vi "ChangeData.vi"(2 "data":string="\"§¶C54ÍÀì6#D\u000b\u00033Ã\u0014ð©À\u0002°B\u0000\u0000\u0000\u0000\u0000\u0000\u0000\u0000\u0006\u0000\u0000\u0000\u0000\u0000\u0010\u0000", 3 "type":string="é\u0003") -> (0 "out":string[][](array[string]), 1 "Contents":string)   [LabVIEW 2018]
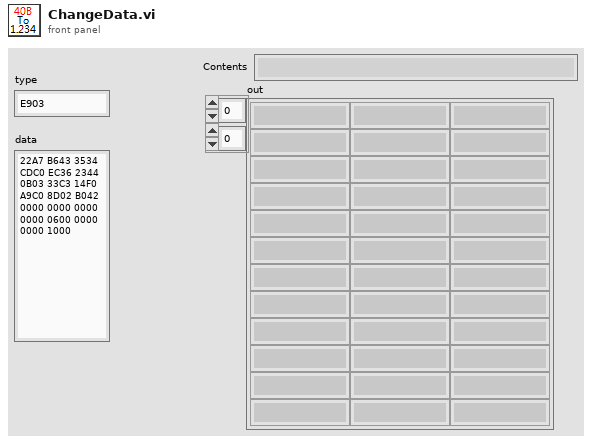
[diagram p1: front panel]
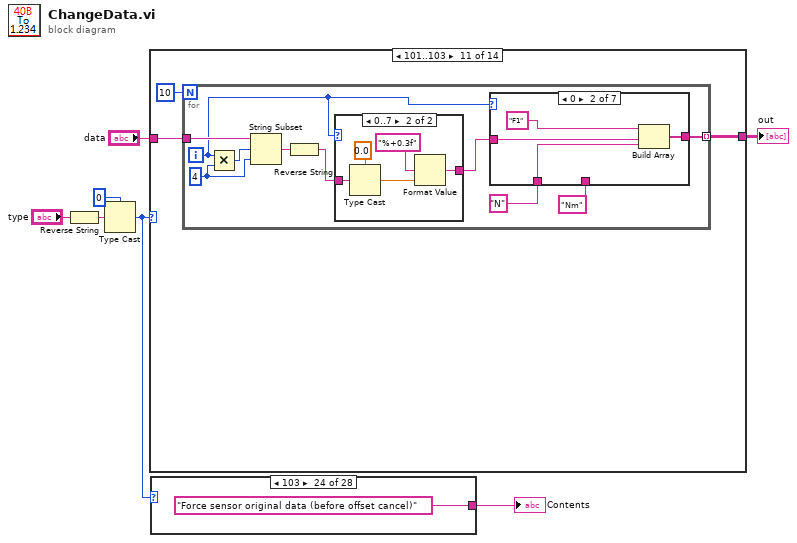
[diagram p0: block diagram]
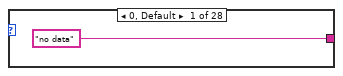
[diagram p2: hidden frame]
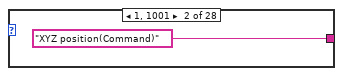
[diagram p3: hidden frame]
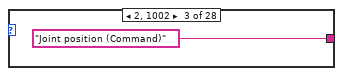
[diagram p4: hidden frame]
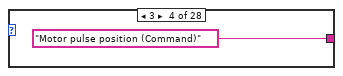
[diagram p5: hidden frame]
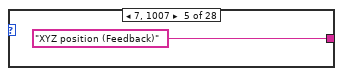
[diagram p6: hidden frame]
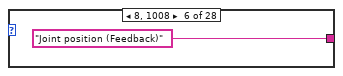
[diagram p7: hidden frame]
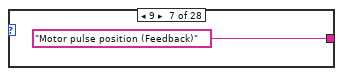
[diagram p8: hidden frame]
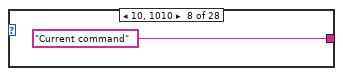
[diagram p9: hidden frame]
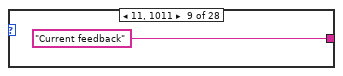
[diagram p10: hidden frame]
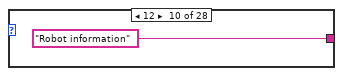
[diagram p11: hidden frame]
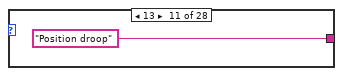
[diagram p12: hidden frame]
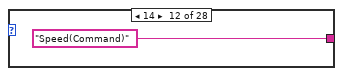
[diagram p13: hidden frame]
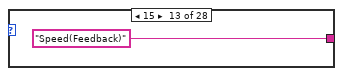
[diagram p14: hidden frame]
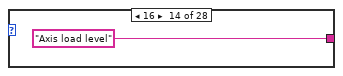
[diagram p15: hidden frame]
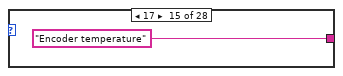
[diagram p16: hidden frame]
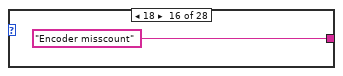
[diagram p17: hidden frame]
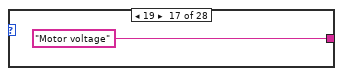
[diagram p18: hidden frame]
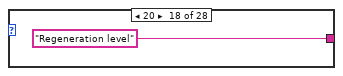
[diagram p19: hidden frame]
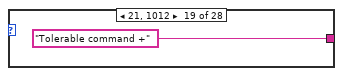
[diagram p20: hidden frame]
diagram:
  n1 = Reverse String(1:"type") -> (0:w7:string)
  n2 = Type Cast(type=u16 0, x=w7) -> (*(type *) &x=w3:u16)
  n3 = case shown="101..103" w3 {
    tunnel: "data" -> [_ w10 w81 w133 w185 w239 w299 w394 w446 w498 w530 w575 w646 w698]
    tunnel: [string[][] [] w9 w80 w132 w184 w238 w322 w393 w445 w497 w529 w574 w645 w697] -> w1
    frame 0, Default {
    }
    frame 1, 7 {
      n4 = for {
        N: 10 -> [_]
        tunnel: w10 -> [w21]
        tunnel: [w17] -> w9 mode=indexing
        i -> [w14]
        w18 = 4
        n5 = Multiply(x=w14, y=w18) -> (x*y=w20:i32)
        n6 = String Subset(string=w21, offset (0)=w20, length (rest)=w18) -> (substring=w19:string)
        n7 = Reverse String(1:w19) -> (0:w16:string)
        n8 = case shown="0..7" w14 {
          tunnel: w16 -> [w22 w24 w31 w36]
          tunnel: [w22 w23 w28 w33] -> w15
          frame -1, Default {
          }
          frame 0..7 {
            n9 = Type Cast(type=sgl 0.0, x=w24) -> (*(type *) &x=w26:sgl)
            n10 = Format Value(format string="%+0.3f", value (0)=w26) -> (output string=w23:string)  [unwired: 1 in]
          }
          frame 8 {
            n11 = Type Cast(type=u32 0, x=w31) -> (*(type *) &x=w30:u32)
            n12 = Format Value(format string="B%08b" ("格式字符串"), value (0)=w30) -> (output string=w28:string)  [unwired: 1 in]
          }
          frame 9 {
            n13 = Type Cast(type=u32 0, x=w36) -> (*(type *) &x=w35:u32)
            n14 = Format Value(format string="H%08x" ("格式字符串"), value (0)=w35) -> (output string=w33:string)  [unwired: 1 in]
          }
        }
        n15 = case shown="8" w14 {
          tunnel: w15 -> [_ w42 w46 w50 w54 w58 w62 w66 w70 w74 w78]
          tunnel: [w38 w41 w45 w49 w53 w57 w61 w64 w68 w72 w76] -> w17
          tunnel: "mm" -> [_ w40 w44 w48 _ _ _ _ _ _ _]
          tunnel: "rad" -> [_ _ _ _ w52 w56 w60 _ _ _ _]
          frame -1, Default {
            w39 = ""
            n16 = Build Array(w39, w39, w39) -> (w38:string[])
          }
          frame 0 {
            n17 = Build Array("X", w42, w40) -> (w41:string[])
          }
          frame 1 {
            n18 = Build Array("Y", w46, w44) -> (w45:string[])
          }
          frame 2 {
            n19 = Build Array("Z", w50, w48) -> (w49:string[])
          }
          frame 3 {
            n20 = Build Array("A", w54, w52) -> (w53:string[])
          }
          frame 4 {
            n21 = Build Array("B", w58, w56) -> (w57:string[])
          }
          frame 5 {
            n22 = Build Array("C", w62, w60) -> (w61:string[])
          }
          frame 6 {
            n23 = Build Array("L1", w66, "") -> (w64:string[])
          }
          frame 7 {
            n24 = Build Array("L2", w70, "") -> (w68:string[])
          }
          frame 8 {
            n25 = Build Array("FL1", w74, "") -> (w72:string[])
          }
          frame 9 {
            n26 = Build Array("FL2", w78, "") -> (w76:string[])
          }
        }
      }
    }
    frame 2, 8 {
      n27 = for {
        N: 10 -> [_]
        tunnel: w81 -> [w91]
        tunnel: [w87] -> w80 mode=indexing
        i -> [w84]
        w88 = 4
        n28 = Multiply(x=w84, y=w88) -> (x*y=w90:i32)
        n29 = String Subset(string=w91, offset (0)=w90, length (rest)=w88) -> (substring=w89:string)
        n30 = Reverse String(1:w89) -> (0:w86:string)
        n31 = case shown="0..7" w84 {
          tunnel: w86 -> [_ w94]
          tunnel: ["" w93] -> w85
          frame -1, Default {
          }
          frame 0..7 {
            n32 = Type Cast(type=sgl 0.0, x=w94) -> (*(type *) &x=w96:sgl)
            n33 = Format Value(format string="%+0.3f", value (0)=w96) -> (output string=w93:string)  [unwired: 1 in]
          }
        }
        n34 = case shown="0" w84 {
          tunnel: w85 -> [_ w102 w106 w110 w114 w118 w122 w126 w130]
          tunnel: [w98 w101 w107 w109 w113 w117 w121 w125 w129] -> w87
          tunnel: "rad" -> [_ w100 w104 w108 w112 w116 w120 w124 w128]
          frame -1, Default {
            w99 = ""
            n35 = Build Array(w99, w99, w99) -> (w98:string[])
          }
          frame 0 {
            n36 = Build Array("J1", w102, w100) -> (w101:string[])
          }
          frame 1 {
            n37 = Build Array("J2", w106, w104) -> (w107:string[])
          }
          frame 2 {
            n38 = Build Array("J3", w110, w108) -> (w109:string[])
          }
          frame 3 {
            n39 = Build Array("J4", w114, w112) -> (w113:string[])
          }
          frame 4 {
            n40 = Build Array("J5", w118, w116) -> (w117:string[])
          }
          frame 5 {
            n41 = Build Array("J6", w122, w120) -> (w121:string[])
          }
          frame 6 {
            n42 = Build Array("J7", w126, w124) -> (w125:string[])
          }
          frame 7 {
            n43 = Build Array("J8", w130, w128) -> (w129:string[])
          }
        }
      }
    }
    frame 3, 9, 13, 18 {
      n44 = for {
        N: 10 -> [_]
        tunnel: w133 -> [w143]
        tunnel: [w139] -> w132 mode=indexing
        i -> [w136]
        w140 = 4
        n45 = Multiply(x=w136, y=w140) -> (x*y=w142:i32)
        n46 = String Subset(string=w143, offset (0)=w142, length (rest)=w140) -> (substring=w141:string)
        n47 = Reverse String(1:w141) -> (0:w138:string)
        n48 = case shown="0..7" w136 {
          tunnel: w138 -> [_ w146]
          tunnel: ["" w145] -> w137
          frame -1, Default {
          }
          frame 0..7 {
            n49 = Type Cast(type=0, x=w146) -> (*(type *) &x=w148:i32)
            n50 = Format Value(format string="%+d", value (0)=w148) -> (output string=w145:string)  [unwired: 1 in]
          }
        }
        n51 = case shown="0" w136 {
          tunnel: w137 -> [_ w154 w158 w162 w166 w170 w174 w178 w182]
          tunnel: [w150 w153 w157 w161 w165 w169 w173 w177 w181] -> w139
          tunnel: "pulse" -> [_ w152 w156 w160 w164 w168 w172 w176 w180]
          frame -1, Default {
            w151 = ""
            n52 = Build Array(w151, w151, w151) -> (w150:string[])
          }
          frame 0 {
            n53 = Build Array("M1", w154, w152) -> (w153:string[])
          }
          frame 1 {
            n54 = Build Array("M2", w158, w156) -> (w157:string[])
          }
          frame 2 {
            n55 = Build Array("M3", w162, w160) -> (w161:string[])
          }
          frame 3 {
            n56 = Build Array("M4", w166, w164) -> (w165:string[])
          }
          frame 4 {
            n57 = Build Array("M5", w170, w168) -> (w169:string[])
          }
          frame 5 {
            n58 = Build Array("M6", w174, w172) -> (w173:string[])
          }
          frame 6 {
            n59 = Build Array("M7", w178, w176) -> (w177:string[])
          }
          frame 7 {
            n60 = Build Array("M8", w182, w180) -> (w181:string[])
          }
        }
      }
    }
    frame 10, 11, 21..23, 111..113 {
      n61 = for {
        N: 10 -> [_]
        tunnel: w185 -> [w195]
        tunnel: [w191] -> w184 mode=indexing
        i -> [w188]
        w192 = 4
        n62 = Multiply(x=w188, y=w192) -> (x*y=w194:i32)
        n63 = String Subset(string=w195, offset (0)=w194, length (rest)=w192) -> (substring=w193:string)
        n64 = Reverse String(1:w193) -> (0:w190:string)
        n65 = case shown="0..7" w188 {
          tunnel: w190 -> [_ w201]
          tunnel: ["" w200] -> w189
          frame -1, Default {
          }
          frame 0..7 {
            n66 = Type Cast(type=0, x=w201) -> (*(type *) &x=w199:i32)
            n67 = Divide(x=w199, y=10.0) -> (x/y=w197:dbl)
            n68 = Format Value(format string="%0.1f", value (0)=w197) -> (output string=w200:string)  [unwired: 1 in]
          }
        }
        n69 = case shown="0" w188 {
          tunnel: w189 -> [_ w208 w212 w216 w220 w224 w228 w232 w236]
          tunnel: [w204 w207 w211 w215 w219 w223 w227 w231 w235] -> w191
          tunnel: "%" -> [_ w206 w210 w214 w218 w222 w226 w230 w234]
          frame -1, Default {
            w205 = ""
            n70 = Build Array(w205, w205, w205) -> (w204:string[])
          }
          frame 0 {
            n71 = Build Array("M1", w208, w206) -> (w207:string[])
          }
          frame 1 {
            n72 = Build Array("M2", w212, w210) -> (w211:string[])
          }
          frame 2 {
            n73 = Build Array("M3", w216, w214) -> (w215:string[])
          }
          frame 3 {
            n74 = Build Array("M4", w220, w218) -> (w219:string[])
          }
          frame 4 {
            n75 = Build Array("M5", w224, w222) -> (w223:string[])
          }
          frame 5 {
            n76 = Build Array("M6", w228, w226) -> (w227:string[])
          }
          frame 6 {
            n77 = Build Array("M7", w232, w230) -> (w231:string[])
          }
          frame 7 {
            n78 = Build Array("M8", w236, w234) -> (w235:string[])
          }
        }
      }
    }
    frame 14, 15 {
      n79 = for {
        N: 10 -> [_]
        tunnel: w239 -> [w249]
        tunnel: [w245] -> w238 mode=indexing
        i -> [w242]
        w246 = 4
        n80 = Multiply(x=w242, y=w246) -> (x*y=w248:i32)
        n81 = String Subset(string=w249, offset (0)=w248, length (rest)=w246) -> (substring=w247:string)
        n82 = Reverse String(1:w247) -> (0:w244:string)
        n83 = case shown="0..7" w242 {
          tunnel: w244 -> [_ w253]
          tunnel: ["" w252] -> w243
          frame -1, Default {
          }
          frame 0..7 {
            n84 = Type Cast(type=0, x=w253) -> (*(type *) &x=w251:i32)
            n85 = Format Value(format string="%d", value (0)=w251) -> (output string=w252:string)  [unwired: 1 in]
          }
        }
        n86 = case shown="0" w242 {
          tunnel: w243 -> [_ w260 w264 w268 w272 w276 w280 w284 w288]
          tunnel: [w256 w259 w263 w267 w271 w275 w279 w283 w287] -> w245
          tunnel: "rpm" -> [_ w258 w262 w266 w270 w274 w278 w282 w286]
          frame -1, Default {
            w257 = ""
            n87 = Build Array(w257, w257, w257) -> (w256:string[])
          }
          frame 0 {
            n88 = Build Array("M1", w260, w258) -> (w259:string[])
          }
          frame 1 {
            n89 = Build Array("M2", w264, w262) -> (w263:string[])
          }
          frame 2 {
            n90 = Build Array("M3", w268, w266) -> (w267:string[])
          }
          frame 3 {
            n91 = Build Array("M4", w272, w270) -> (w271:string[])
          }
          frame 4 {
            n92 = Build Array("M5", w276, w274) -> (w275:string[])
          }
          frame 5 {
            n93 = Build Array("M6", w280, w278) -> (w279:string[])
          }
          frame 6 {
            n94 = Build Array("M7", w284, w282) -> (w283:string[])
          }
          frame 7 {
            n95 = Build Array("M8", w288, w286) -> (w287:string[])
          }
        }
      }
    }
    frame 12 {
      n96 = for {
        N: 5 -> [_]
        tunnel: w299 -> [w370]
        tunnel: [w366] -> w324 mode=indexing
        i -> [w363]
        w367 = 4
        n97 = Multiply(x=w363, y=w367) -> (x*y=w369:i32)
        n98 = String Subset(string=w370, offset (0)=w369, length (rest)=w367) -> (substring=w368:string)
        n99 = Reverse String(1:w368) -> (0:w365:string)
        n100 = Type Cast(type=0, x=w365) -> (*(type *) &x=w360:i32)
        n101 = Format Value(format string="%d", value (0)=w360) -> (output string=w364:string)  [unwired: 1 in]
        n102 = case shown="0" w363 {
          tunnel: w364 -> [_ w375 w379 w383 w387 w391]
          tunnel: [w371 w374 w378 w382 w386 w390] -> w366
          frame -1, Default {
            w372 = ""
            n103 = Build Array(w372, w372, w372) -> (w371:string[])
          }
          frame 0 {
            n104 = Build Array("Tool point speed(feedback)", w375, "mm/s") -> (w374:string[])
          }
          frame 1 {
            n105 = Build Array("Remaining distance(feedback)", w379, "mm") -> (w378:string[])
          }
          frame 2 {
            n106 = Build Array("Tool point speed(Command)", w383, "mm/s") -> (w382:string[])
          }
          frame 3 {
            n107 = Build Array("Remaining distance(Command)", w387, "mm") -> (w386:string[])
          }
          frame 4 {
            n108 = Build Array("Gap of command and feedback", w391, "") -> (w390:string[])
          }
        }
      }
      n109 = String Subset(string=w299, offset (0)=20 ("偏移量(0)"), length (rest)=6 ("长度（剩余）")) -> (substring=w326:string)
      n110 = String Subset(string=w299, offset (0)=26 ("偏移量(0)"), length (rest)=6 ("长度（剩余）")) -> (substring=w319:string)
      n111 = String Subset(string=w299, offset (0)=32 ("偏移量(0)"), length (rest)=2 ("长度（剩余）")) -> (substring=w312:string)
      n112 = String Subset(string=w299, offset (0)=36 ("偏移量(0)"), length (rest)=4 ("长度（剩余）")) -> (substring=w298:string)
      n113 = for {
        N: 3 -> [_]
        tunnel: w326 -> [w334]
        tunnel: [w330] -> w323 mode=indexing
        i -> [w332]
        w333 = 2
        n114 = Multiply(x=w332, y=w333) -> (x*y=w336:i32)
        n115 = String Subset(string=w334, offset (0)=w336, length (rest)=w333) -> (substring=w337:string)
        n116 = Reverse String(1:w337) -> (0:w338:string)
        n117 = Type Cast(type=i16 0, x=w338) -> (*(type *) &x=w340:i16)
        n118 = Format Value(format string="%d", value (0)=w340) -> (output string=w331:string)  [unwired: 1 in]
        n119 = case shown="2" w332 {
          tunnel: w331 -> [_ w345 w348 w358]
          tunnel: [w341 w343 w349 w356] -> w330
          frame -1, Default {
            w342 = ""
            n120 = Build Array(w342, w342, w342) -> (w341:string[])
          }
          frame 0 {
            n121 = Build Array("Transport factor (command)", w345, "") -> (w343:string[])
          }
          frame 1 {
            n122 = case shown="\"假\", 默认" w348 {
              tunnel: ["" "Stopped" "Accelerating" "Constant speed" "Decelerating"] -> w347
              frame "假", Default {
              }
              frame "0" {
              }
              frame "1" {
              }
              frame "2" {
              }
              frame "3" {
              }
            }
            n123 = Build Array("Acceleration state(command)", w348, w347) -> (w349:string[])
          }
          frame 2 {
            n124 = Build Array("Step number( slot 1)", w358, "") -> (w356:string[])
          }
        }
      }
      n125 = Reverse String(1:w298) -> (0:w297:string)
      n126 = Reverse String(1:w319) -> (0:w316:string)
      n127 = Reverse String(1:w312) -> (0:w311:string)
      n128 = Type Cast(type=0, x=w297) -> (*(type *) &x=w295:i32)
      n129 = Type Cast(type=i16 0, x=w311) -> (*(type *) &x=w309:i16)
      n130 = Divide(x=w309, y=i16 10) -> (x/y=w307:dbl)
      n131 = Format Value(format string="%d", value (0)=w295) -> (output string=w291:string)  [unwired: 1 in]
      n132 = Format Value(format string="%0.1f", value (0)=w307) -> (output string=w303:string)  [unwired: 1 in]
      n133 = Build Array("Program name( slot 1)", w316, "") -> (w315:string[])
      n134 = Build Array("Monitoring counter", w291, "X 7.1ms") -> (w290:string[])
      n135 = Build Array("Controller temperature", w303, "℃") -> (w302:string[])
      n136 = Build Array (concatenate)(w324, w323, w315, w302, w290) -> (w322:string[][])
    }
    frame 16, 20 {
      n137 = for {
        N: 10 -> [_]
        tunnel: w394 -> [w404]
        tunnel: [w400] -> w393 mode=indexing
        i -> [w397]
        w401 = 4
        n138 = Multiply(x=w397, y=w401) -> (x*y=w403:i32)
        n139 = String Subset(string=w404, offset (0)=w403, length (rest)=w401) -> (substring=w402:string)
        n140 = Reverse String(1:w402) -> (0:w399:string)
        n141 = case shown="0..7" w397 {
          tunnel: w399 -> [_ w408]
          tunnel: ["" w407] -> w398
          frame -1, Default {
          }
          frame 0..7 {
            n142 = Type Cast(type=sgl 0.0, x=w408) -> (*(type *) &x=w406:sgl)
            n143 = Format Value(format string="%0.3f", value (0)=w406) -> (output string=w407:string)  [unwired: 1 in]
          }
        }
        n144 = case shown="0" w397 {
          tunnel: w398 -> [_ w415 w419 w423 w427 w431 w435 w439 w443]
          tunnel: [w411 w414 w418 w422 w426 w430 w434 w438 w442] -> w400
          tunnel: "%" -> [_ w413 w417 w421 w425 w429 w433 w437 w441]
          frame -1, Default {
            w412 = ""
            n145 = Build Array(w412, w412, w412) -> (w411:string[])
          }
          frame 0 {
            n146 = Build Array("M1", w415, w413) -> (w414:string[])
          }
          frame 1 {
            n147 = Build Array("M2", w419, w417) -> (w418:string[])
          }
          frame 2 {
            n148 = Build Array("M3", w423, w421) -> (w422:string[])
          }
          frame 3 {
            n149 = Build Array("M4", w427, w425) -> (w426:string[])
          }
          frame 4 {
            n150 = Build Array("M5", w431, w429) -> (w430:string[])
          }
          frame 5 {
            n151 = Build Array("M6", w435, w433) -> (w434:string[])
          }
          frame 6 {
            n152 = Build Array("M7", w439, w437) -> (w438:string[])
          }
          frame 7 {
            n153 = Build Array("M8", w443, w441) -> (w442:string[])
          }
        }
      }
    }
    frame 17 {
      n154 = for {
        N: 10 -> [_]
        tunnel: w446 -> [w456]
        tunnel: [w452] -> w445 mode=indexing
        i -> [w449]
        w453 = 4
        n155 = Multiply(x=w449, y=w453) -> (x*y=w455:i32)
        n156 = String Subset(string=w456, offset (0)=w455, length (rest)=w453) -> (substring=w454:string)
        n157 = Reverse String(1:w454) -> (0:w451:string)
        n158 = case shown="0..7" w449 {
          tunnel: w451 -> [_ w460]
          tunnel: ["" w459] -> w450
          frame -1, Default {
          }
          frame 0..7 {
            n159 = Type Cast(type=0, x=w460) -> (*(type *) &x=w458:i32)
            n160 = Format Value(format string="%d", value (0)=w458) -> (output string=w459:string)  [unwired: 1 in]
          }
        }
        n161 = case shown="0" w449 {
          tunnel: w450 -> [_ w467 w471 w475 w479 w483 w487 w491 w495]
          tunnel: [w463 w466 w470 w474 w478 w482 w486 w490 w494] -> w452
          tunnel: "℃" -> [_ w465 w469 w473 w477 w481 w485 w489 w493]
          frame -1, Default {
            w464 = ""
            n162 = Build Array(w464, w464, w464) -> (w463:string[])
          }
          frame 0 {
            n163 = Build Array("M1", w467, w465) -> (w466:string[])
          }
          frame 1 {
            n164 = Build Array("M2", w471, w469) -> (w470:string[])
          }
          frame 2 {
            n165 = Build Array("M3", w475, w473) -> (w474:string[])
          }
          frame 3 {
            n166 = Build Array("M4", w479, w477) -> (w478:string[])
          }
          frame 4 {
            n167 = Build Array("M5", w483, w481) -> (w482:string[])
          }
          frame 5 {
            n168 = Build Array("M6", w487, w485) -> (w486:string[])
          }
          frame 6 {
            n169 = Build Array("M7", w491, w489) -> (w490:string[])
          }
          frame 7 {
            n170 = Build Array("M8", w495, w493) -> (w494:string[])
          }
        }
      }
    }
    frame 19 {
      n171 = for {
        N: 10 -> [_]
        tunnel: w498 -> [w508]
        tunnel: [w504] -> w497 mode=indexing
        i -> [w501]
        w505 = 4
        n172 = Multiply(x=w501, y=w505) -> (x*y=w507:i32)
        n173 = String Subset(string=w508, offset (0)=w507, length (rest)=w505) -> (substring=w506:string)
        n174 = Reverse String(1:w506) -> (0:w503:string)
        n175 = case shown="0..2" w501 {
          tunnel: w503 -> [_ w512]
          tunnel: ["" w511] -> w502
          frame -1, Default {
          }
          frame 0..2 {
            n176 = Type Cast(type=0, x=w512) -> (*(type *) &x=w510:i32)
            n177 = Format Value(format string="%d", value (0)=w510) -> (output string=w511:string)  [unwired: 1 in]
          }
        }
        n178 = case shown="2" w501 {
          tunnel: w502 -> [_ w519 w523 w527]
          tunnel: [w515 w518 w522 w526] -> w504
          tunnel: "V" -> [_ w517 w521 w525]
          frame -1, Default {
            w516 = ""
            n179 = Build Array(w516, w516, w516) -> (w515:string[])
          }
          frame 0 {
            n180 = Build Array("Motor power voltage", w519, w517) -> (w518:string[])
          }
          frame 1 {
            n181 = Build Array("Motor power voltage(MAX)", w523, w521) -> (w522:string[])
          }
          frame 2 {
            n182 = Build Array("Motor power voltage(MIN)", w527, w525) -> (w526:string[])
          }
        }
      }
    }
    frame 101..103 {
      n183 = for {
        N: 10 -> [_]
        tunnel: w530 -> [w541]
        tunnel: [w537] -> w529 mode=indexing
        i -> [w534]
        w538 = 4
        n184 = Multiply(x=w534, y=w538) -> (x*y=w540:i32)
        n185 = String Subset(string=w541, offset (0)=w540, length (rest)=w538) -> (substring=w539:string)
        n186 = Reverse String(1:w539) -> (0:w536:string)
        n187 = case shown="0..7" w534 {
          tunnel: w536 -> [_ w545]
          tunnel: ["" w544] -> w535
          frame -1, Default {
          }
          frame 0..7 {
            n188 = Type Cast(type=0.0, x=w545) -> (*(type *) &x=w543:dbl)
            n189 = Format Value(format string="%+0.3f", value (0)=w543) -> (output string=w544:string)  [unwired: 1 in]
          }
        }
        n190 = case shown="0" w534 {
          tunnel: w535 -> [_ w552 w556 w560 w564 w568 w572]
          tunnel: [w548 w551 w555 w559 w563 w567 w571] -> w537
          tunnel: "N" -> [_ w550 w554 w558 _ _ _]
          tunnel: "Nm" -> [_ _ _ _ w562 w566 w570]
          frame -1, Default {
            w549 = ""
            n191 = Build Array(w549, w549, w549) -> (w548:string[])
          }
          frame 0 {
            n192 = Build Array("F1", w552, w550) -> (w551:string[])
          }
          frame 1 {
            n193 = Build Array("F2", w556, w554) -> (w555:string[])
          }
          frame 2 {
            n194 = Build Array("F3", w560, w558) -> (w559:string[])
          }
          frame 3 {
            n195 = Build Array("F4", w564, w562) -> (w563:string[])
          }
          frame 4 {
            n196 = Build Array("F5", w568, w566) -> (w567:string[])
          }
          frame 5 {
            n197 = Build Array("F6", w572, w570) -> (w571:string[])
          }
        }
      }
    }
    frame 1001, 1007 {
      n198 = for {
        N: 10 -> [_]
        tunnel: w575 -> [w586]
        tunnel: [w582] -> w574 mode=indexing
        i -> [w579]
        w583 = 4
        n199 = Multiply(x=w579, y=w583) -> (x*y=w585:i32)
        n200 = String Subset(string=w586, offset (0)=w585, length (rest)=w583) -> (substring=w584:string)
        n201 = Reverse String(1:w584) -> (0:w581:string)
        n202 = case shown="0..7" w579 {
          tunnel: w581 -> [w587 w589 w596 w601]
          tunnel: [w587 w588 w593 w598] -> w580
          frame -1, Default {
          }
          frame 0..7 {
            n203 = Type Cast(type=sgl 0.0, x=w589) -> (*(type *) &x=w591:sgl)
            n204 = Format Value(format string="%+0.3f", value (0)=w591) -> (output string=w588:string)  [unwired: 1 in]
          }
          frame 8 {
            n205 = Type Cast(type=u32 0, x=w596) -> (*(type *) &x=w595:u32)
            n206 = Format Value(format string="B%08b" ("格式字符串"), value (0)=w595) -> (output string=w593:string)  [unwired: 1 in]
          }
          frame 9 {
            n207 = Type Cast(type=u32 0, x=w601) -> (*(type *) &x=w600:u32)
            n208 = Format Value(format string="H%08x" ("格式字符串"), value (0)=w600) -> (output string=w598:string)  [unwired: 1 in]
          }
        }
        n209 = case shown="5" w579 {
          tunnel: w580 -> [_ w607 w611 w615 w619 w623 w627 w631 w635 w639 w643]
          tunnel: [w603 w606 w610 w614 w618 w622 w626 w629 w633 w637 w641] -> w582
          tunnel: "mm" -> [_ w605 w609 w613 _ _ _ _ _ _ _]
          tunnel: "deg" -> [_ _ _ _ w617 w621 w625 _ _ _ _]
          frame -1, Default {
            w604 = ""
            n210 = Build Array(w604, w604, w604) -> (w603:string[])
          }
          frame 0 {
            n211 = Build Array("X", w607, w605) -> (w606:string[])
          }
          frame 1 {
            n212 = Build Array("Y", w611, w609) -> (w610:string[])
          }
          frame 2 {
            n213 = Build Array("Z", w615, w613) -> (w614:string[])
          }
          frame 3 {
            n214 = Build Array("A", w619, w617) -> (w618:string[])
          }
          frame 4 {
            n215 = Build Array("B", w623, w621) -> (w622:string[])
          }
          frame 5 {
            n216 = Build Array("C", w627, w625) -> (w626:string[])
          }
          frame 6 {
            n217 = Build Array("L1", w631, "") -> (w629:string[])
          }
          frame 7 {
            n218 = Build Array("L2", w635, "") -> (w633:string[])
          }
          frame 8 {
            n219 = Build Array("FL1", w639, "") -> (w637:string[])
          }
          frame 9 {
            n220 = Build Array("FL2", w643, "") -> (w641:string[])
          }
        }
      }
    }
    frame 1002, 1008 {
      n221 = for {
        N: 10 -> [_]
        tunnel: w646 -> [w656]
        tunnel: [w652] -> w645 mode=indexing
        i -> [w649]
        w653 = 4
        n222 = Multiply(x=w649, y=w653) -> (x*y=w655:i32)
        n223 = String Subset(string=w656, offset (0)=w655, length (rest)=w653) -> (substring=w654:string)
        n224 = Reverse String(1:w654) -> (0:w651:string)
        n225 = case shown="0..7" w649 {
          tunnel: w651 -> [_ w659]
          tunnel: ["" w658] -> w650
          frame -1, Default {
          }
          frame 0..7 {
            n226 = Type Cast(type=sgl 0.0, x=w659) -> (*(type *) &x=w661:sgl)
            n227 = Format Value(format string="%+0.3f", value (0)=w661) -> (output string=w658:string)  [unwired: 1 in]
          }
        }
        n228 = case shown="3" w649 {
          tunnel: w650 -> [_ w667 w671 w675 w679 w683 w687 w691 w695]
          tunnel: [w663 w666 w672 w674 w678 w682 w686 w690 w694] -> w652
          tunnel: "deg" -> [_ w665 w669 w673 w677 w681 w685 w689 w693]
          frame -1, Default {
            w664 = ""
            n229 = Build Array(w664, w664, w664) -> (w663:string[])
          }
          frame 0 {
            n230 = Build Array("J1", w667, w665) -> (w666:string[])
          }
          frame 1 {
            n231 = Build Array("J2", w671, w669) -> (w672:string[])
          }
          frame 2 {
            n232 = Build Array("J3", w675, w673) -> (w674:string[])
          }
          frame 3 {
            n233 = Build Array("J4", w679, w677) -> (w678:string[])
          }
          frame 4 {
            n234 = Build Array("J5", w683, w681) -> (w682:string[])
          }
          frame 5 {
            n235 = Build Array("J6", w687, w685) -> (w686:string[])
          }
          frame 6 {
            n236 = Build Array("J7", w691, w689) -> (w690:string[])
          }
          frame 7 {
            n237 = Build Array("J8", w695, w693) -> (w694:string[])
          }
        }
      }
    }
    frame 1010..1014 {
      n238 = for {
        N: 10 -> [_]
        tunnel: w698 -> [w708]
        tunnel: [w704] -> w697 mode=indexing
        i -> [w701]
        w705 = 4
        n239 = Multiply(x=w701, y=w705) -> (x*y=w707:i32)
        n240 = String Subset(string=w708, offset (0)=w707, length (rest)=w705) -> (substring=w706:string)
        n241 = Reverse String(1:w706) -> (0:w703:string)
        n242 = case shown="0..7" w701 {
          tunnel: w703 -> [_ w712]
          tunnel: ["" w711] -> w702
          frame -1, Default {
          }
          frame 0..7 {
            n243 = Type Cast(type=sgl 0.0, x=w712) -> (*(type *) &x=w710:sgl)
            n244 = Format Value(format string="%0.3f", value (0)=w710) -> (output string=w711:string)  [unwired: 1 in]
          }
        }
        n245 = case shown="0" w701 {
          tunnel: w702 -> [_ w719 w723 w727 w731 w735 w739 w743 w747]
          tunnel: [w715 w718 w722 w726 w730 w734 w738 w742 w746] -> w704
          tunnel: "A" -> [_ w717 w721 w725 w729 w733 w737 w741 w745]
          frame -1, Default {
            w716 = ""
            n246 = Build Array(w716, w716, w716) -> (w715:string[])
          }
          frame 0 {
            n247 = Build Array("M1", w719, w717) -> (w718:string[])
          }
          frame 1 {
            n248 = Build Array("M2", w723, w721) -> (w722:string[])
          }
          frame 2 {
            n249 = Build Array("M3", w727, w725) -> (w726:string[])
          }
          frame 3 {
            n250 = Build Array("M4", w731, w729) -> (w730:string[])
          }
          frame 4 {
            n251 = Build Array("M5", w735, w733) -> (w734:string[])
          }
          frame 5 {
            n252 = Build Array("M6", w739, w737) -> (w738:string[])
          }
          frame 6 {
            n253 = Build Array("M7", w743, w741) -> (w742:string[])
          }
          frame 7 {
            n254 = Build Array("M8", w747, w745) -> (w746:string[])
          }
        }
      }
    }
  }
  "out" <- w1
  n255 = case shown="103" w3 {
    tunnel: ["no data" "XYZ position(Command)" "Joint position (Command)" "Motor pulse position (Command)" "XYZ position (Feedback)" "Joint position (Feedback)" "Motor pulse position (Feedback)" "Current command" "Current feedback" "Robot information" "Position droop" "Speed(Command)" "Speed(Feedback)" "Axis load level" "Encoder temperature" "Encoder misscount" "Motor voltage" "Regeneration level" "Tolerable command +" "Tolerable command -" "RMS current" "Force sensor current position" "Force sensor original data (after offset cancel) " "Force sensor original data (before offset cancel)" "Position command of the force sensor correction" "COL presumed torque" "COL threshold + " "COL threshold - "] -> w2
    frame 0, Default {
    }
    frame 1, 1001 {
    }
    frame 2, 1002 {
    }
    frame 3 {
    }
    frame 7, 1007 {
    }
    frame 8, 1008 {
    }
    frame 9 {
    }
    frame 10, 1010 {
    }
    frame 11, 1011 {
    }
    frame 12 {
    }
    frame 13 {
    }
    frame 14 {
    }
    frame 15 {
    }
    frame 16 {
    }
    frame 17 {
    }
    frame 18 {
    }
    frame 19 {
    }
    frame 20 {
    }
    frame 21, 1012 {
    }
    frame 22, 1013 {
    }
    frame 23, 1014 {
    }
    frame 101 {
    }
    frame 102 {
    }
    frame 103 {
    }
    frame 104 {
    }
    frame 111 {
    }
    frame 112 {
    }
    frame 113 {
    }
  }
  "Contents" <- w2
